vi "Load Pattern Core.vi"(8 "error in (no error)":errorcluster, 10 "PatternData":T1(array[cluster]), 11 "CS++PPG in":refnum<class "CS++PPG.lvclass">) -> (0 "error out":errorcluster, 3 "CS++PPG out":refnum<class "CS++PPG.lvclass">)   [LabVIEW 2016, in "CS++PPG.lvlib" / "CS++PPG.lvclass"]
doc: "This VI loads a pattern to the pulsed pattern generator. Afterwards the PPG device should be ready to start."
uses:
  CS++PPG.lvclass
  CS++PPG.lvclass/CS++PPG.ctl
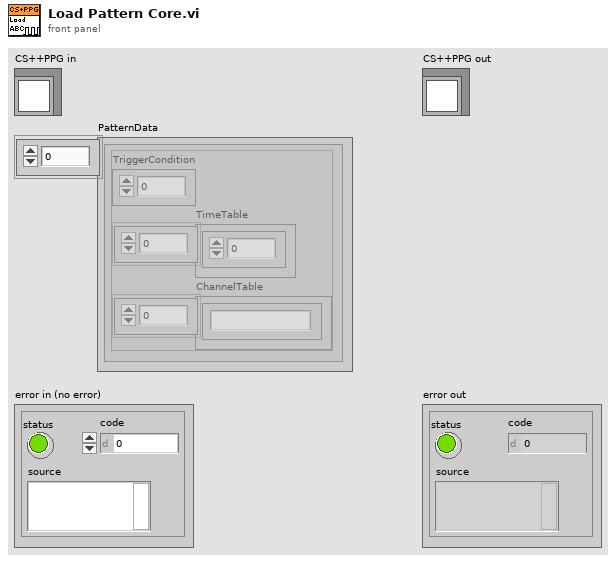
[diagram p1: front panel]
types:
  T1 = cluster{"TriggerCondition":i32, "TimeTable":dbl[], "ChannelTable":string[]}[]
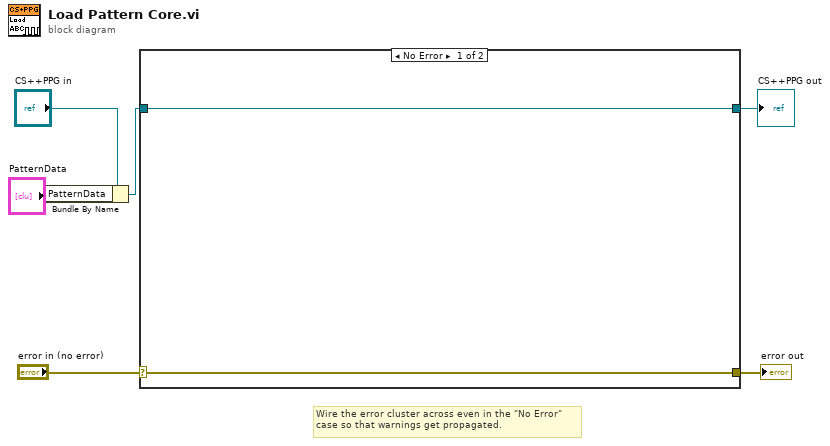
[diagram p0: block diagram]
diagram:
  # "Wire the error cluster across even in the \"No Error\"\ncase so that warnings get propagated."
  n1 = Bundle By Name(cluster="CS++PPG in", "PatternData"="PatternData") -> (w1:refnum<class "CS++PPG.lvclass">)
  n2 = case shown="No Error" "error in (no error)" {
    selector: "error in (no error)" -> [w8 w10]
    tunnel: [w8 w10] -> w5
    tunnel: [w7 w9] -> w4
    tunnel: w1 -> [w7 w9]
    frame No Error {
    }
    frame Error {
    }
  }
  "error out" <- w5
  "CS++PPG out" <- w4
